vi "_attribute_write_int32.vi"(5 "Repeated Capability":string, 7 "Attribute":T1={"Identifier"="", "Descriptive Name"="", "Data Type"=enum."Integer 32", "Command"="", "Access"=enum."Read/Write", "Range Table"="", "Read Callback"="", "Write Callback"="", "Supported Models"="", "Instrument Options"="", "Index"=0, "OPC Wait"=FALSE, "No Status Check"=FALSE, "Cache Only"=FALSE}, 8 "error in":errorcluster caption="error in (no error)", 10 "Int32 in":i32, 11 "VISA resource name":refnum<visa-resource-name>) -> (0 "error out":errorcluster, 3 "VISA resource name out":refnum<visa-resource-name>)   [LabVIEW 2020, in "Rohde&Schwarz RTx Oscilloscopes.lvlib" / "rsidr_core.lvlib"]
uses:
  rsidr_core.lvlib
  type_Attribute.ctl
  type_Attribute_Data_Type.ctl
  type_ReadWriteAccess.ctl
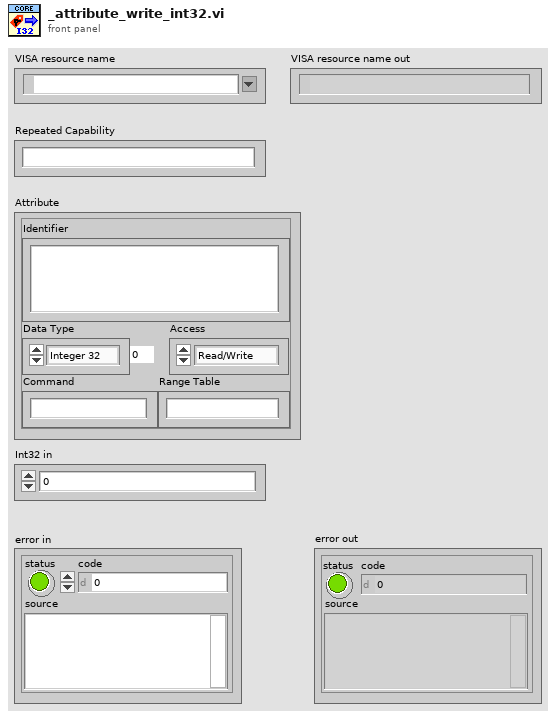
[diagram p1: front panel]
types:
  T1 = typedef "Rohde&Schwarz RTx Oscilloscopes.lvlib/rsidr_core.lvlib/type_Attribute.ctl" = cluster{"Identifier":string, "Descriptive Name":string, "Data Type":T2, "Command":string, "Access":T3, "Range Table":string, "Read Callback":string, "Write Callback":string, "Supported Models":string, "Instrument Options":string, "Index":i32, "OPC Wait":bool, "No Status Check":bool, "Cache Only":bool}
  T2 = typedef "Rohde&Schwarz RTx Oscilloscopes.lvlib/rsidr_core.lvlib/type_Attribute_Data_Type.ctl" = enum16{"Integer 32", "Double", "String", "Boolean", "None", "Integer 64", "RawString"}
  T3 = typedef "Rohde&Schwarz RTx Oscilloscopes.lvlib/rsidr_core.lvlib/type_ReadWriteAccess.ctl" = enum16{"Read Only", "Write Only", "Read/Write"}
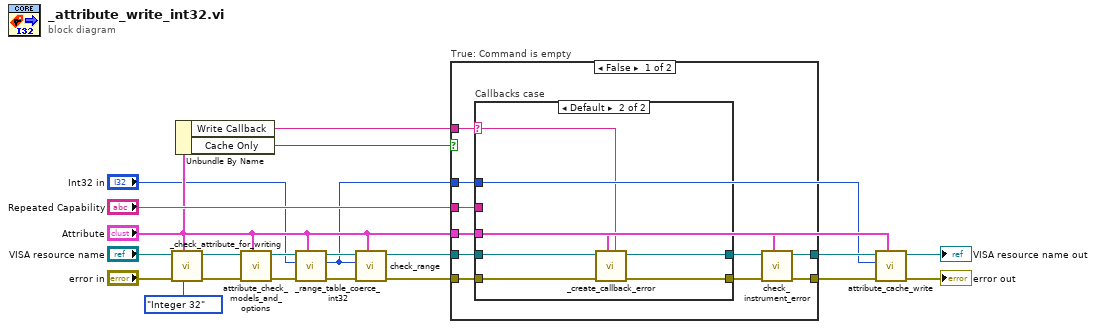
[diagram p0: block diagram]
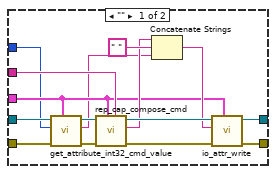
[diagram p2: hidden frame]
diagram:
  n1 = call "_check_attribute_for_writing.vi"("Expected Data Type"=type_Attribute_Data_Type."Integer 32" ("Data Type"), "Attribute"="Attribute", "error in"="error in", "VISA resource name"="VISA resource name") -> ("error out"=w8:errorcluster, "VISA resource name out"=w7:refnum<visa-resource-name>)  [unwired: 6 in]
  n2 = Unbundle By Name("Attribute") -> ("Write Callback"=w15:string, "Cache Only"=w1:bool)
  n3 = call "attribute_check_models_and_options.vi"("Attribute"="Attribute", "error in"=w8, "VISA resource name"=w7) -> ("error out"=w6:errorcluster, "VISA resource name out"=w5:refnum<visa-resource-name>)  [unwired: 6 in, 1 out]
  n4 = call "_range_table_coerce_int32.vi"("Attribute"="Attribute", "error in"=w6, "Int32 in"="Int32 in", "VISA resource name"=w5) -> ("error out"=w14:errorcluster, "Int32 out"=w2:i32, "VISA resource name out"=w13:refnum<visa-resource-name>)  [unwired: 5 in]
  n5 = call "check_range.vi"("Attribute"="Attribute", "error in"=w14, "Value to check"=w2, "VISA resource name"=w13) -> ("error out"=w12:errorcluster, "VISA resource name out"=w11:refnum<visa-resource-name>)  [unwired: 6 in]
  n6 = case "True: Command is empty" shown="False" w1 {
    tunnel: "Repeated Capability" -> [w31 _]
    tunnel: w12 -> [w30 w53]
    tunnel: w11 -> [w29 w54]
    tunnel: w2 -> [w28 _]
    tunnel: "Attribute" -> [w22 _]
    tunnel: [w23 w54] -> w9
    tunnel: [w24 w53] -> w10
    tunnel: w15 -> [w27 _]
    frame False {
      n7 = case "Callbacks case" shown="Default" w27 {
        selector: w27 -> [_ w47]
        tunnel: w28 -> [w33 _]
        tunnel: w29 -> [w37 w51]
        tunnel: w30 -> [w38 w52]
        tunnel: w31 -> [w42 _]
        tunnel: [w44 w49] -> w25
        tunnel: [w43 w50] -> w26
        tunnel: w22 -> [w34 w48]
        frame "" {
          n8 = call "get_attribute_int32_cmd_value.vi"("Attribute"=w34, "error in"=w38, "Input Int32 value"=w33, "VISA resource name"=w37) -> ("error out"=w36:errorcluster, "Cmd Value out"=w32:string, "VISA resource name out"=w35:refnum<visa-resource-name>)  [unwired: 5 in]
          n9 = call "rep_cap_compose_cmd.vi"("Repeated Capability"=w42, "Attribute"=w34, "error in"=w36, "VISA resource name"=w35) -> ("error out"=w45:errorcluster, "Command out"=w39:string, "VISA resource name out"=w46:refnum<visa-resource-name>)  [unwired: 5 in]
          n10 = Concatenate Strings(w39, " ", w32) -> (w40:string)
          n11 = call "io_attr_write.vi"("Attribute"=w34, "error in"=w45, "write buffer"=w40, "VISA resource name"=w46) -> ("error out"=w43:errorcluster, "VISA resource name out"=w44:refnum<visa-resource-name>)  [unwired: 6 in]
        }
        frame Default {
          n12 = call "_create_callback_error.vi"("Callback Name"=w47, "Attribute"=w48, "error in"=w52, "VISA resource name"=w51) -> ("error out"=w50:errorcluster, "VISA resource name out"=w49:refnum<visa-resource-name>)  [unwired: 6 in]
        }
      }
      n13 = call "check_instrument_error.vi"("Attribute"=w22, "error in"=w26, "VISA resource name"=w25) -> ("error out"=w24:errorcluster, "VISA resource name out"=w23:refnum<visa-resource-name>)  [unwired: 7 in]
    }
    frame True {
    }
  }
  n14 = call "attribute_cache_write.vi"("Attribute"="Attribute", "error in"=w10, "Value in"=w2, "VISA resource name"=w9) -> ("error out"=→"error out":errorcluster, "VISA resource name out"=→"VISA resource name out":refnum<visa-resource-name>)  [unwired: 6 in]
